vi "PH_Synchrolock_Watch.show History.vi"(0 "i ref in":refnum<vi>, 5 "error in":errorcluster) -> (14 "i ref out":refnum<vi>, 19 "error out":errorcluster)   [LabVIEW 2014, in "PH_Synchrolock_Watch.lvlib"]
doc: "This VI shows the result including the previous in graphs."
uses:
  PH_Synchrolock_Watch.lvlib
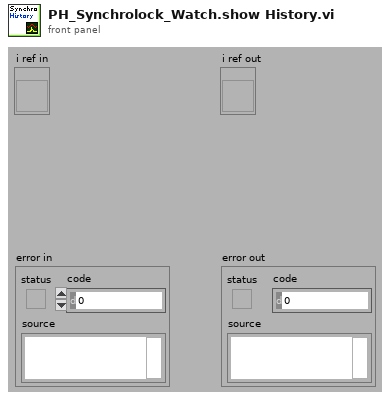
[diagram p1: front panel]
types:
  T1 = typedef "PH_Synchrolock_Watch.lvlib/PH_Synchrolock_Watch.i attribute.ctl" = cluster{"GUI Refs":cluster{"Mean Phase Graph":refnum<vi>, "RF Amplitude Graph":refnum<vi>, "Mira Amplitude Graph":refnum<vi>, "MIRA State":refnum<vi>, "Mean Phase":refnum<vi>, "RF Amplitude":refnum<vi>, "Mira Amplitude":refnum<vi>, "Mean Phase in range?":refnum<vi>, "RF Amplitude above limit?":refnum<vi>, "Mira Amplitude in range?":refnum<vi>, "Mean phase upper limit":refnum<vi>, "Mean phase lower limit":refnum<vi>, "RF Amplitude lower limit":refnum<vi>, "Mira Amplitude lower limit":refnum<vi>, "Mira Amplitude upper limit":refnum<vi>, "Mira scope":refnum<vi>, "Reset Mira warning":refnum<vi>}, "Status":cluster{"Reset Warning":bool}, "Mean Phase":cluster{"Current Value":dbl, "Upper Limit":dbl, "Lower Limit":dbl, "Data":cluster{dbl[], dbl[]}}, "RF":cluster{"Current Value":dbl, "Lower Limit":dbl, "Data":cluster{dbl[], dbl[]}}, "MIRA":cluster{"Current Value":dbl, "Upper Limit":dbl, "Lower Limit":dbl, "Data":cluster{dbl[], dbl[]}}}
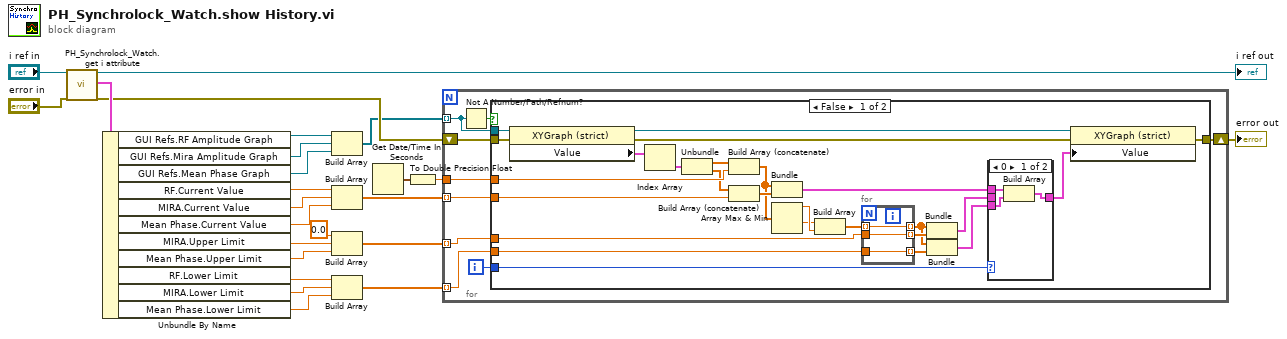
[diagram p0: block diagram]
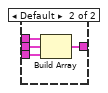
[diagram p2: hidden frame]
diagram:
  n1 = call "PH_Synchrolock_Watch.get i attribute.vi"("i ref in"="i ref in", "error in (no error)"="error in") -> ("i ref out"=→"i ref out":refnum<vi>, "i attribute"=w24:T1, "error out"=w22:errorcluster)  [unwired: 15 in]
  n2 = Unbundle By Name(w24) -> ("GUI Refs.RF Amplitude Graph"=w17:refnum<vi>, "GUI Refs.Mira Amplitude Graph"=w16:refnum<vi>, "GUI Refs.Mean Phase Graph"=w15:refnum<vi>, "RF.Current Value"=w12:dbl, "MIRA.Current Value"=w11:dbl, "Mean Phase.Current Value"=w10:dbl, "MIRA.Upper Limit"=w7:dbl, "Mean Phase.Upper Limit"=w6:dbl, "RF.Lower Limit"=w8:dbl, "MIRA.Lower Limit"=w5:dbl, "Mean Phase.Lower Limit"=w4:dbl)
  n3 = Build Array(w17, w16, w15) -> (w14:refnum<vi>[])
  n4 = Build Array(w12, w11, w10) -> (w9:dbl[])
  n5 = Build Array(0.0 ("element"), w7, w6) -> (w2:dbl[])
  n6 = Build Array(w8, w5, w4) -> (w1:dbl[])
  n7 = Get Date/Time In Seconds() -> (seconds since 1Jan1904=w18:timestamp)
  n8 = To Double Precision Float(number=w18) -> (double precision float=w13:dbl)
  n9 = for {
    shift-right: [w33] -> w19
    shift-left: w22 -> [w30]
    tunnel: w14 -> [w31] mode=indexing
    tunnel: w13 -> [w29]
    tunnel: w9 -> [w28] mode=indexing
    tunnel: w2 -> [w27] mode=indexing
    tunnel: w1 -> [w26] mode=indexing
    i -> [w25]
    n10 = Not A Number/Path/Refnum?(number/path/refnum=w31) -> (NaN/Path/Refnum?=w32:bool)
    n11 = case shown="False" w32 {
      tunnel: w30 -> [w59 w70]
      tunnel: [w48 w70] -> w33
      tunnel: w31 -> [w58 _]
      tunnel: w29 -> [w54 _]
      tunnel: w28 -> [w52 _]
      tunnel: w27 -> [w39 _]
      tunnel: w26 -> [w38 _]
      tunnel: w25 -> [w34 _]
      frame False {
        n12 = property class="XYGraph (strict)"(reference=w58, error in=w59) -> (reference out=w47:refnum<vi>, error out=w49:errorcluster, "Value"=w57:cluster{dbl[], dbl[]}[])
        n13 = Index Array(array=w57) -> (element=w56:cluster{dbl[], dbl[]})  [unwired: 1 in]
        n14 = Unbundle(w56) -> (w55:dbl[], w53:dbl[])
        n15 = Build Array (concatenate)(w55, w54) -> (w40:dbl[])
        n16 = Build Array (concatenate)(w53, w52) -> (w51:dbl[])
        n17 = Bundle(w40, w51) -> (w50:cluster{dbl[], dbl[]})  [unwired: 1 in]
        n18 = Array Max & Min(array=w40) -> (max value=w45:dbl, min value=w41:dbl)  [unwired: 2 out]
        n19 = Build Array(w41, w45) -> (w42:dbl[])
        n20 = for {
          tunnel: w42 -> [w68] mode=indexing
          tunnel: w39 -> [w69]
          tunnel: [w69] -> w43 mode=indexing
          tunnel: [w68] -> w37 mode=indexing
          tunnel: w38 -> [w67]
          tunnel: [w67] -> w44 mode=indexing
        }
        n21 = Bundle(w37, w43) -> (w36:cluster{dbl[], dbl[]})  [unwired: 1 out]
        n22 = Bundle(w37, w44) -> (w35:cluster{dbl[], dbl[]})  [unwired: 1 out]
        n23 = case shown="0" w34 {
          tunnel: w50 -> [w62 w66]
          tunnel: [w61 w65] -> w46
          tunnel: w36 -> [_ w64]
          tunnel: w35 -> [w60 w63]
          frame 0 {
            n24 = Build Array(w62, w60) -> (w61:cluster{dbl[], dbl[]}[])
          }
          frame Default {
            n25 = Build Array(w66, w64, w63) -> (w65:cluster{dbl[], dbl[]}[])
          }
        }
        n26 = property class="XYGraph (strict)"(reference=w47, error in=w49, "Value"=w46) -> (error out=w48:errorcluster)  [unwired: 1 out]
      }
      frame True {
      }
    }
  }
  "error out" <- w19
